vi "Recieve Result.vi"(8 "error in (no error)":errorcluster, 10 "Mag Lab Result.lvclass":refnum<class "Mag Lab Result.lvclass">, 11 "Cap Bank Idot Measurement in":refnum<class "Cap Bank Idot Measurement.lvclass">) -> (0 "error out":errorcluster, 3 "Cap Bank Idot Measurement out":refnum<class "Cap Bank Idot Measurement.lvclass">)   [LabVIEW 2012, in "Cap Bank Idot Measurement.lvclass"]
uses:
  Cap Bank Idot Measurement.lvclass
  Mag Lab Result/Mag Lab Result.lvclass
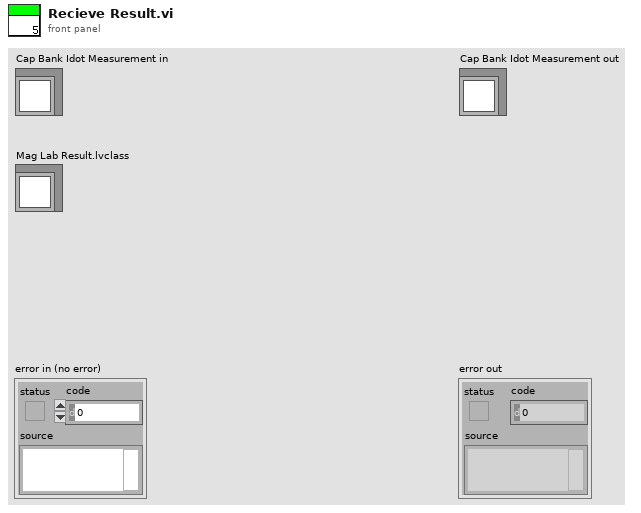
[diagram p1: front panel]
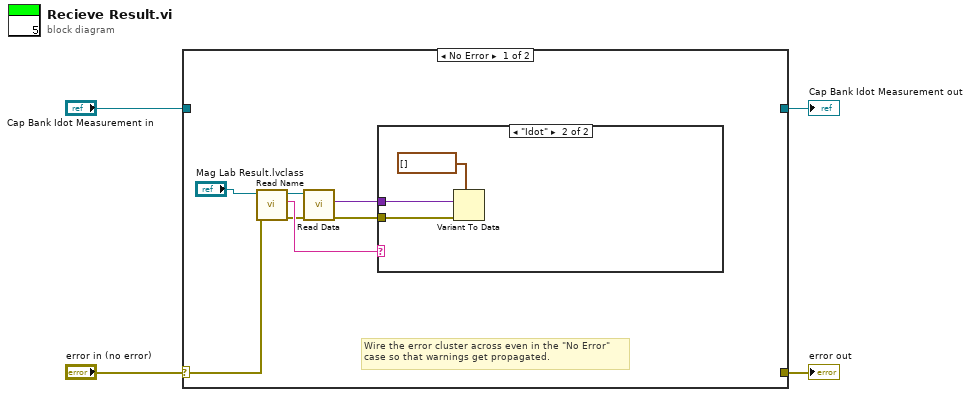
[diagram p0: block diagram]
diagram:
  n1 = case shown="No Error" "error in (no error)" {
    selector: "error in (no error)" -> [w9 w16]
    tunnel: [_ w16] -> w3
    tunnel: [_ w15] -> w1
    tunnel: "Cap Bank Idot Measurement in" -> [_ w15]
    frame No Error {
      # "Wire the error cluster across even in the \"No Error\"\ncase so that warnings get propagated."
      n2 = call "Read Name.vi"("error in (no error)"=w9, "Mag Lab Result in"="Mag Lab Result.lvclass") -> ("error out"=w5:errorcluster, "Name"=w10:string, "Mag Lab Result out"=w8:refnum<class "Mag Lab Result.lvclass">)  [unwired: 7 in]
      n3 = call "Read Data.vi"("error in (no error)"=w5, "Mag Lab Result in"=w8) -> ("error out"=w6:errorcluster, "Data"=w7:variant)  [unwired: 7 in, 1 out]
      n4 = case shown="\"Idot\"" w10 {
        tunnel: w7 -> [_ w13]
        tunnel: w6 -> [_ w12]
        frame "\u0000", Default {
        }
        frame "Idot" {
          n5 = Variant To Data(error in=w12, type=waveform(dbl)[] [] ("data"), Variant=w13) -> ()  [unwired: 2 out]
        }
      }
    }
    frame Error {
    }
  }
  "error out" <- w3
  "Cap Bank Idot Measurement out" <- w1
